vi "PrintExcel.vi"() -> ()   [LabVIEW 2011]
uses:
  <vilib>/Utility/NIReport.llb/NI_report.lvclass
  <vilib>/addons/_office/NI_ReportGenerationToolkit.lvlib
panel:
  in  "uL温度":string[](array[string])
  in  "IL温度":string[](array[string])
  in  "uL电流系数":string[](array[string])
  in  "IL电流系数":string[](array[string])
  in  "curRange":string
  in  "MLFB":string
  in  "Voltage":dbl[](array[numeric])
  in  "KG uL":dbl[](array[numeric])
  in  "KG IL":dbl[](array[numeric])
  in  "Trip uL":i32[](array[numeric])
  in  "Trip IL":i32[](array[numeric])
  in  "start(-1,-1)":cluster{"row":i32, "column":i32}
  in  "report file path":path
  out "error out":errorcluster
  in  "template (empty)":path
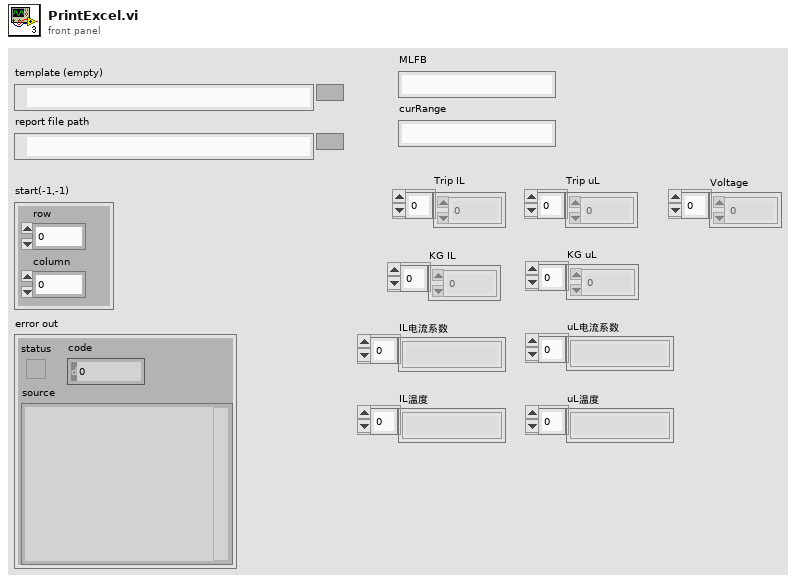
[diagram p1: front panel]
types:
  T1 = enum16{"maximized", "minimized", "normal", "no change"}
  T2 = enum16{"Standard Report", "HTML", "Word", "Excel"}
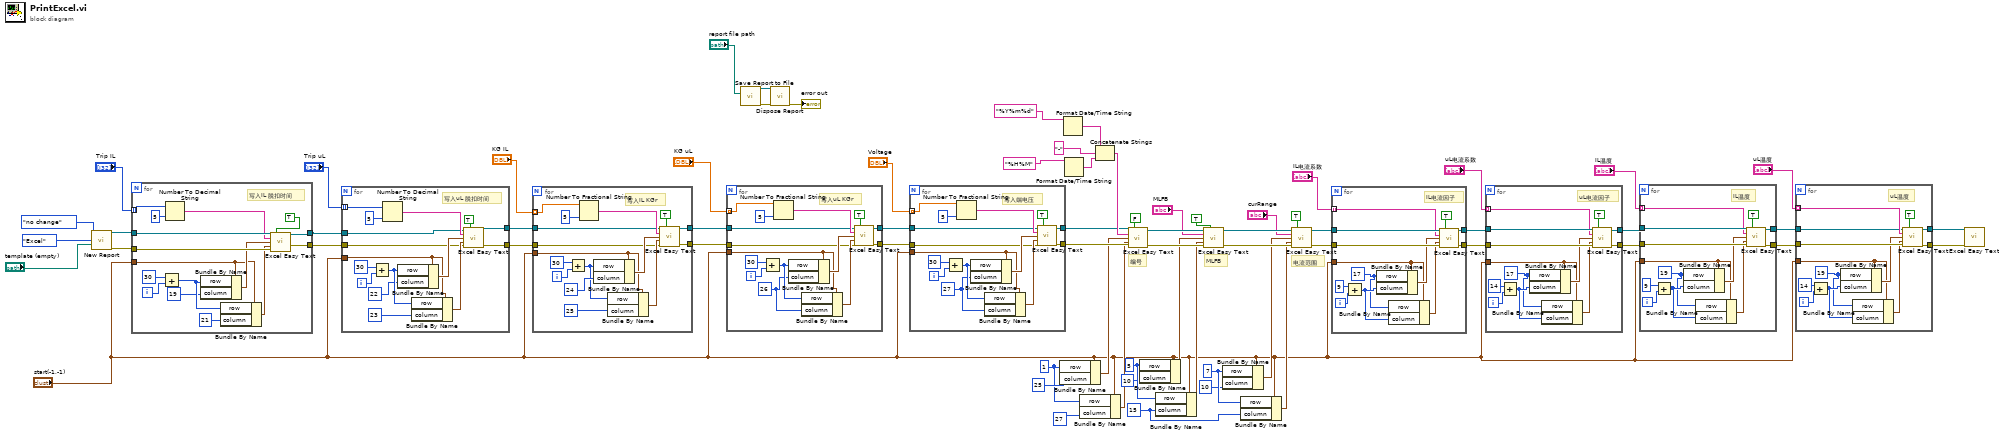
[diagram p0: block diagram]
diagram:
  w20 = 7 ("row")
  w18 = 15 ("column")
  w28 = 5 ("row")
  w29 = 1 ("row")
  # "编号"
  # "电流范围"
  # "MLFB"
  n1 = call <vilib>:"New Report.vi"("window state (normal)"=T1."no change", "report type"=T2."Excel", "template (empty)"="template (empty)") -> ("report out"=w66:refnum<class "NI_report.lvclass">, "error out"=w65:errorcluster)  [unwired: 11 in]
  n2 = for {
    tunnel: w66 -> [w84]
    tunnel: w65 -> [w83]
    tunnel: [w82] -> w58
    tunnel: [w81] -> w57
    tunnel: "start(-1,-1)" -> [w69]
    tunnel: "Trip IL" -> [w73] mode=indexing
    i -> [w76]
    # "写入IL 脱扣时间"
    n3 = Add(x=30, y=w76) -> (x+y=w77:i32)
    n4 = Number To Decimal String(number=w73, width (-)=i16 5) -> (decimal integer string=w71:string)
    n5 = Bundle By Name(cluster=w69, "row"=w77, "column"=19 ("x")) -> (w80:cluster{"row":i32, "column":i32})
    n6 = Bundle By Name(cluster=w69, "row"=w77, "column"=21) -> (w79:cluster{"row":i32, "column":i32})
    n7 = call <vilib>:"Excel Easy Text.vi"("report in"=w84, "border? (F)"=TRUE, "text"=w71, "start (-1, -1)"=w80, "end (-1, -1)"=w79, "error in (no error)"=w83) -> ("report out"=w82:refnum<class "NI_report.lvclass">, "error out"=w81:errorcluster)  [unwired: 5 in, 3 out]
  }
  n8 = for {
    tunnel: w58 -> [w88]
    tunnel: w57 -> [w87]
    tunnel: "Trip uL" -> [w98] mode=indexing
    tunnel: "start(-1,-1)" -> [w95]
    tunnel: [w86] -> w54
    tunnel: [w85] -> w53
    i -> [w92]
    # "写入uL 脱扣时间"
    n9 = Add(x=30 ("row"), y=w92) -> (x+y=w91:i32)
    n10 = Number To Decimal String(number=w98, width (-)=i16 5) -> (decimal integer string=w97:string)
    n11 = Bundle By Name(cluster=w95, "row"=w91, "column"=22) -> (w96:cluster{"row":i32, "column":i32})
    n12 = Bundle By Name(cluster=w95, "row"=w91, "column"=23) -> (w94:cluster{"row":i32, "column":i32})
    n13 = call <vilib>:"Excel Easy Text.vi"("report in"=w88, "border? (F)"=TRUE, "text"=w97, "start (-1, -1)"=w96, "end (-1, -1)"=w94, "error in (no error)"=w87) -> ("report out"=w86:refnum<class "NI_report.lvclass">, "error out"=w85:errorcluster)  [unwired: 5 in, 3 out]
  }
  n14 = for {
    tunnel: "KG IL" -> [w103] mode=indexing
    tunnel: "start(-1,-1)" -> [w106]
    tunnel: w54 -> [w105]
    tunnel: w53 -> [w104]
    tunnel: [w102] -> w51
    tunnel: [w101] -> w50
    i -> [w107]
    # "写入IL KGr"
    n15 = Add(x=30 ("row"), y=w107) -> (x+y=w114:i32)
    n16 = Number To Fractional String(number=w103, precision (6)=i16 5 ("width (-)")) -> (F-format string=w110:string)  [unwired: 2 in]
    n17 = Bundle By Name(cluster=w106, "row"=w114, "column"=24) -> (w111:cluster{"row":i32, "column":i32})
    n18 = Bundle By Name(cluster=w106, "row"=w114, "column"=25) -> (w112:cluster{"row":i32, "column":i32})
    n19 = call <vilib>:"Excel Easy Text.vi"("report in"=w105, "border? (F)"=TRUE, "text"=w110, "start (-1, -1)"=w111, "end (-1, -1)"=w112, "error in (no error)"=w104) -> ("report out"=w102:refnum<class "NI_report.lvclass">, "error out"=w101:errorcluster)  [unwired: 5 in, 3 out]
  }
  n20 = for {
    tunnel: "KG uL" -> [w121] mode=indexing
    tunnel: "start(-1,-1)" -> [w123]
    tunnel: w50 -> [w122]
    tunnel: w51 -> [w120]
    tunnel: [w119] -> w48
    tunnel: [w118] -> w47
    i -> [w124]
    w117 = 26 ("column")
    # "写入uL KGr"
    n21 = Add(x=30 ("row"), y=w124) -> (x+y=w131:i32)
    n22 = Number To Fractional String(number=w121, precision (6)=i16 5 ("width (-)")) -> (F-format string=w127:string)  [unwired: 2 in]
    n23 = Bundle By Name(cluster=w123, "row"=w131, "column"=w117) -> (w128:cluster{"row":i32, "column":i32})
    n24 = Bundle By Name(cluster=w123, "row"=w131, "column"=w117) -> (w129:cluster{"row":i32, "column":i32})
    n25 = call <vilib>:"Excel Easy Text.vi"("report in"=w120, "border? (F)"=TRUE, "text"=w127, "start (-1, -1)"=w128, "end (-1, -1)"=w129, "error in (no error)"=w122) -> ("report out"=w119:refnum<class "NI_report.lvclass">, "error out"=w118:errorcluster)  [unwired: 5 in, 3 out]
  }
  n26 = call-dynamic "Save Report to File.vi"("report file path"="report file path") -> ("report out"=w64:refnum<class "NI_report.lvclass">, "error out"=w63:errorcluster)  [unwired: 13 in]
  n27 = call-dynamic "Dispose Report.vi"("report in"=w64, "error in (no error)"=w63) -> ("error out"=→"error out":errorcluster)  [unwired: 13 in]
  n28 = for {
    tunnel: "Voltage" -> [w136] mode=indexing
    tunnel: "start(-1,-1)" -> [w138]
    tunnel: w47 -> [w137]
    tunnel: w48 -> [w135]
    tunnel: [w134] -> w42
    tunnel: [w133] -> w41
    i -> [w139]
    w132 = 27 ("column")
    # "写入端电压"
    n29 = Add(x=30 ("row"), y=w139) -> (x+y=w146:i32)
    n30 = Number To Fractional String(number=w136, precision (6)=i16 5 ("width (-)")) -> (F-format string=w142:string)  [unwired: 2 in]
    n31 = Bundle By Name(cluster=w138, "row"=w146, "column"=w132) -> (w143:cluster{"row":i32, "column":i32})
    n32 = Bundle By Name(cluster=w138, "row"=w146, "column"=w132) -> (w144:cluster{"row":i32, "column":i32})
    n33 = call <vilib>:"Excel Easy Text.vi"("report in"=w135, "border? (F)"=TRUE, "text"=w142, "start (-1, -1)"=w143, "end (-1, -1)"=w144, "error in (no error)"=w137) -> ("report out"=w134:refnum<class "NI_report.lvclass">, "error out"=w133:errorcluster)  [unwired: 5 in, 3 out]
  }
  n34 = Bundle By Name(cluster="start(-1,-1)", "row"=w29, "column"=25) -> (w40:cluster{"row":i32, "column":i32})
  n35 = Format Date/Time String(time format string (%c)="%Y%m%d") -> (date/time string=w46:string)  [unwired: 2 in]
  n36 = Format Date/Time String(time format string (%c)="%H%M") -> (date/time string=w2:string)  [unwired: 2 in]
  n37 = Bundle By Name(cluster="start(-1,-1)", "row"=w29, "column"=27) -> (w37:cluster{"row":i32, "column":i32})
  n38 = Concatenate Strings(w46, "-" ("string"), w2) -> (w43:string)
  n39 = call <vilib>:"Excel Easy Text.vi"("report in"=w42, "border? (F)"=FALSE, "text"=w43, "start (-1, -1)"=w40, "end (-1, -1)"=w37, "error in (no error)"=w41) -> ("report out"=w35:refnum<class "NI_report.lvclass">, "error out"=w34:errorcluster)  [unwired: 5 in, 3 out]
  n40 = Bundle By Name(cluster="start(-1,-1)", "row"=w28, "column"=10) -> (w31:cluster{"row":i32, "column":i32})
  n41 = Bundle By Name(cluster="start(-1,-1)", "row"=w28, "column"=w18) -> (w30:cluster{"row":i32, "column":i32})
  n42 = call <vilib>:"Excel Easy Text.vi"("report in"=w35, "border? (F)"=TRUE, "text"="MLFB", "start (-1, -1)"=w31, "end (-1, -1)"=w30, "error in (no error)"=w34) -> ("report out"=w26:refnum<class "NI_report.lvclass">, "error out"=w25:errorcluster)  [unwired: 5 in, 3 out]
  n43 = Bundle By Name(cluster="start(-1,-1)", "row"=w20, "column"=10) -> (w24:cluster{"row":i32, "column":i32})
  n44 = Bundle By Name(cluster="start(-1,-1)", "row"=w20, "column"=w18) -> (w23:cluster{"row":i32, "column":i32})
  n45 = call <vilib>:"Excel Easy Text.vi"("report in"=w26, "border? (F)"=TRUE, "text"="curRange", "start (-1, -1)"=w24, "end (-1, -1)"=w23, "error in (no error)"=w25) -> ("report out"=w17:refnum<class "NI_report.lvclass">, "error out"=w16:errorcluster)  [unwired: 5 in, 3 out]
  n46 = for {
    tunnel: w17 -> [w159]
    tunnel: w16 -> [w158]
    tunnel: "IL电流系数" -> [w154] mode=indexing
    tunnel: "start(-1,-1)" -> [w152]
    tunnel: [w148] -> w13
    tunnel: [w147] -> w12
    i -> [w151]
    w149 = 17 ("row")
    # "IL电流因子"
    n47 = Add(x=9, y=w151) -> (x+y=w150:i32)
    n48 = Bundle By Name(cluster=w152, "row"=w149, "column"=w150) -> (w155:cluster{"row":i32, "column":i32})
    n49 = Bundle By Name(cluster=w152, "row"=w149, "column"=w150) -> (w156:cluster{"row":i32, "column":i32})
    n50 = call <vilib>:"Excel Easy Text.vi"("report in"=w159, "border? (F)"=TRUE, "text"=w154, "start (-1, -1)"=w155, "end (-1, -1)"=w156, "error in (no error)"=w158) -> ("report out"=w148:refnum<class "NI_report.lvclass">, "error out"=w147:errorcluster)  [unwired: 5 in, 3 out]
  }
  n51 = for {
    tunnel: w13 -> [w172]
    tunnel: w12 -> [w171]
    tunnel: "uL电流系数" -> [w167] mode=indexing
    tunnel: "start(-1,-1)" -> [w165]
    tunnel: [w161] -> w10
    tunnel: [w160] -> w9
    i -> [w164]
    w162 = 17 ("row")
    # "uL电流因子"
    n52 = Add(x=14, y=w164) -> (x+y=w163:i32)
    n53 = Bundle By Name(cluster=w165, "row"=w162, "column"=w163) -> (w168:cluster{"row":i32, "column":i32})
    n54 = Bundle By Name(cluster=w165, "row"=w162, "column"=w163) -> (w169:cluster{"row":i32, "column":i32})
    n55 = call <vilib>:"Excel Easy Text.vi"("report in"=w172, "border? (F)"=TRUE, "text"=w167, "start (-1, -1)"=w168, "end (-1, -1)"=w169, "error in (no error)"=w171) -> ("report out"=w161:refnum<class "NI_report.lvclass">, "error out"=w160:errorcluster)  [unwired: 5 in, 3 out]
  }
  n56 = for {
    tunnel: w10 -> [w185]
    tunnel: w9 -> [w184]
    tunnel: "IL温度" -> [w180] mode=indexing
    tunnel: "start(-1,-1)" -> [w178]
    tunnel: [w174] -> w7
    tunnel: [w173] -> w6
    i -> [w177]
    w175 = 19 ("row")
    # "IL温度"
    n57 = Add(x=9, y=w177) -> (x+y=w176:i32)
    n58 = Bundle By Name(cluster=w178, "row"=w175, "column"=w176) -> (w181:cluster{"row":i32, "column":i32})
    n59 = Bundle By Name(cluster=w178, "row"=w175, "column"=w176) -> (w182:cluster{"row":i32, "column":i32})
    n60 = call <vilib>:"Excel Easy Text.vi"("report in"=w185, "border? (F)"=TRUE, "text"=w180, "start (-1, -1)"=w181, "end (-1, -1)"=w182, "error in (no error)"=w184) -> ("report out"=w174:refnum<class "NI_report.lvclass">, "error out"=w173:errorcluster)  [unwired: 5 in, 3 out]
  }
  n61 = for {
    tunnel: w6 -> [w198]
    tunnel: "uL温度" -> [w194] mode=indexing
    tunnel: "start(-1,-1)" -> [w192]
    tunnel: [w188] -> w4
    tunnel: [w187] -> w3
    tunnel: w7 -> [w186]
    i -> [w191]
    w189 = 19 ("row")
    # "uL温度"
    n62 = Add(x=14, y=w191) -> (x+y=w190:i32)
    n63 = Bundle By Name(cluster=w192, "row"=w189, "column"=w190) -> (w195:cluster{"row":i32, "column":i32})
    n64 = Bundle By Name(cluster=w192, "row"=w189, "column"=w190) -> (w196:cluster{"row":i32, "column":i32})
    n65 = call <vilib>:"Excel Easy Text.vi"("report in"=w186, "border? (F)"=TRUE, "text"=w194, "start (-1, -1)"=w195, "end (-1, -1)"=w196, "error in (no error)"=w198) -> ("report out"=w188:refnum<class "NI_report.lvclass">, "error out"=w187:errorcluster)  [unwired: 5 in, 3 out]
  }
  n66 = call <vilib>:"Excel Easy Text.vi"("report in"=w4, "error in (no error)"=w3) -> ()  [unwired: 9 in, 5 out]
